vi "ReadVariantId.vi"(8 "error in (no error)":errorcluster, 11 "BME68x in":refnum<class "BME680.lvclass">) -> (0 "error out":errorcluster, 3 "BME68x out":refnum<class "BME680.lvclass">)   [LabVIEW 2022 SP3, in "BME680.lvlib" / "BME680.lvclass"]
uses:
  BME680.lvclass
  BME680.lvclass/BME680.ctl
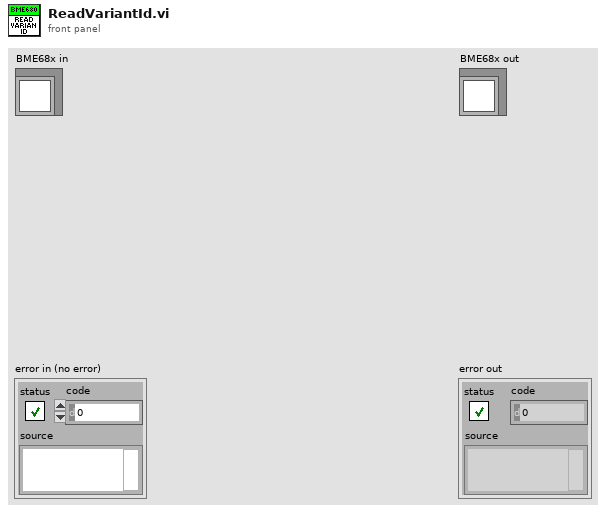
[diagram p1: front panel]
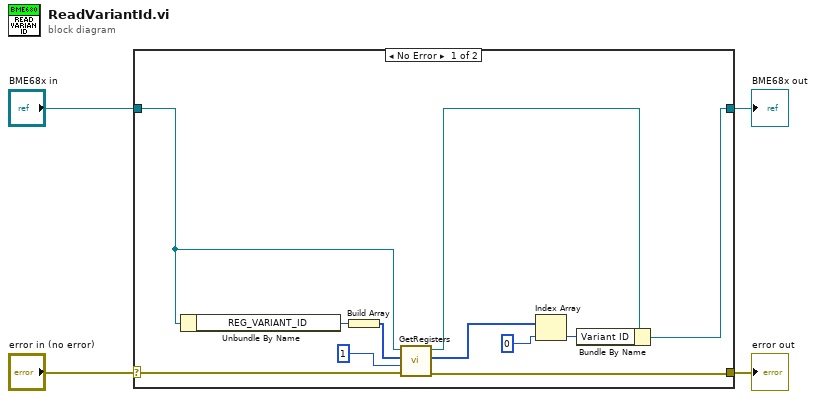
[diagram p0: block diagram]
diagram:
  n1 = case shown="No Error" "error in (no error)" {
    selector: "error in (no error)" -> [w15 w17]
    tunnel: [w14 w17] -> w3
    tunnel: [w6 w16] -> w1
    tunnel: "BME68x in" -> [w13 w16]
    frame No Error {
      n2 = Unbundle By Name(w13) -> ("REG_VARIANT_ID"=w12:u8)
      n3 = Build Array(w12) -> (w11:u8[])
      n4 = call-dynamic "GetRegisters.vi"("error in (no error)"=w15, "Lenght"=u8 1, "Addr"=w11, "BME680 in"=w13) -> ("error out"=w14:errorcluster, "Data out"=w9:u8[], "BME680 out"=w7:refnum<class "BME680.lvclass">)  [unwired: 5 in]
      n5 = Index Array(array=w9, index=0) -> (element=w5:u8)
      n6 = Bundle By Name(cluster=w7, "Variant ID"=w5) -> (w6:refnum<class "BME680.lvclass">)
    }
    frame Error {
    }
  }
  "error out" <- w3
  "BME68x out" <- w1
